vi "ReadNodeClass.vi"(8 "error in":errorcluster, 11 "node in":refnum<class "NISE_CEF_Node.lvclass">) -> (0 "error out":errorcluster, 2 "nodeClass":string, 3 "node out":refnum<class "NISE_CEF_Node.lvclass">)   [LabVIEW 2013, in "NISE_CEF_Node.lvclass"]
uses:
  NISE_CEF_Node.lvclass
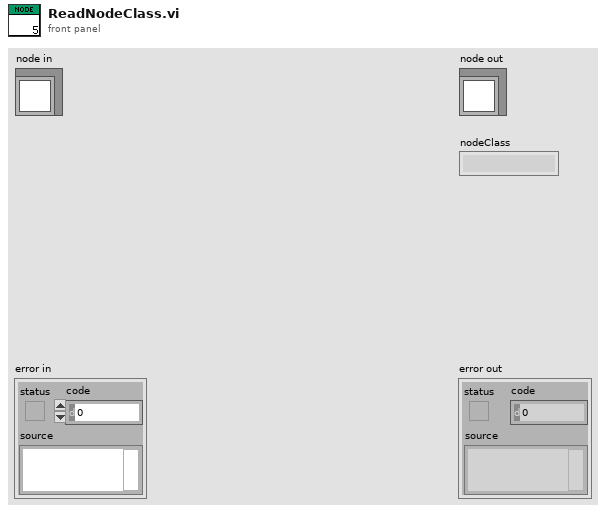
[diagram p1: front panel]
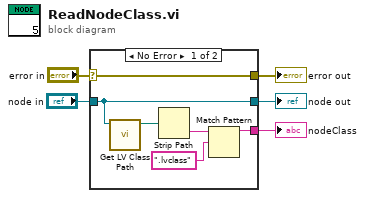
[diagram p0: block diagram]
diagram:
  n1 = case shown="No Error" "error in" {
    selector: "error in" -> [w11 w13]
    tunnel: [w11 w13] -> w4
    tunnel: [w10 w12] -> w2
    tunnel: "node in" -> [w10 w12]
    tunnel: [w6 _] -> w1
    frame No Error {
      n2 = call <vilib>:"Get LV Class Path.vi"("object"=w10) -> ("class path"=w7:path)  [unwired: 9 in, 1 out]
      n3 = Strip Path(path=w7) -> (name=w9:string)  [unwired: 1 out]
      n4 = Match Pattern(string=w9, regular expression=".lvclass") -> (before substring=w6:string)  [unwired: 1 in, 3 out]
    }
    frame Error {
    }
  }
  "error out" <- w4
  "node out" <- w2
  "nodeClass" <- w1
